vi "GetAppInfoInCluster.vi"(0 "Cluster":cluster{"App Refnum":refnum<vi>}) -> (1 "VI Version":string, 2 "Application:User Name":string, 3 "Operating System:Name":string, 4 "error out":errorcluster)   [LabVIEW 2010]
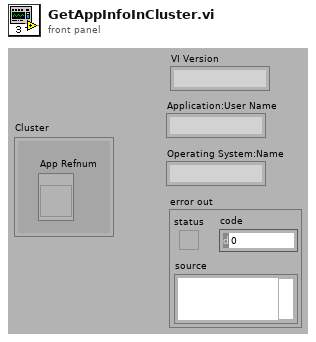
[diagram p1: front panel]
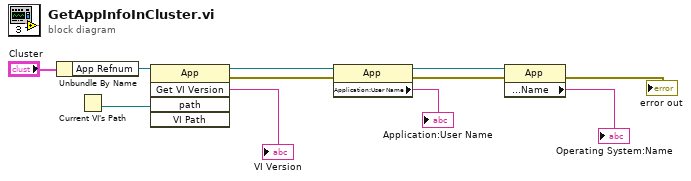
[diagram p0: block diagram]
diagram:
  n1 = Unbundle By Name("Cluster") -> ("App Refnum"=w1:refnum<vi>)
  n2 = Current VI's Path() -> (path=w11:path)
  n3 = invoke class="App" method="Get VI Version"(reference=w1, "path"=w11) -> (reference out=w9:refnum<vi>, error out=w8:errorcluster, "GetVIVers"=→"VI Version":string)  [unwired: 3 in, 2 out]
  n4 = property class="App"(reference=w9, error in=w8) -> (reference out=w7:refnum<vi>, error out=w6:errorcluster, "Application:User Name"=→"Application:User Name":string)
  n5 = property class="App"(reference=w7, error in=w6) -> (error out=→"error out":errorcluster, "Operating System:Name"=→"Operating System:Name":string)  [unwired: 1 out]
